vi "NF WF1973_74 OPER Enab.vi"(6 "Read(F)":bool, 8 "error in (no error)":errorcluster caption="Error IN", 9 "Channel(Unavailable)":u16(ring) items=["Unavailable", "Ch1", "Ch2"], 10 "Event Enable(0)":i32(knob) min=0 max=65535 step=1 scale=0.0..65535.0, 11 "VISAsession":refnum<visa-resource-name>) -> (0 "error out":errorcluster caption="Error OUT", 2 "Query Event Enable":i32=99999, 3 "CopyVISAsession":refnum<visa-resource-name>)   [LabVIEW 2010]
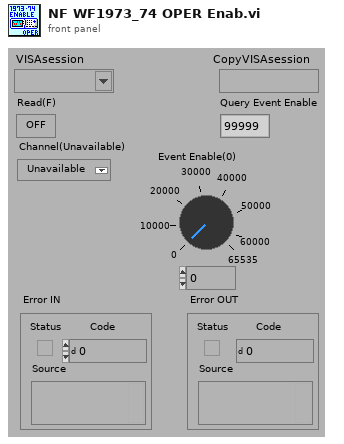
[diagram p1: front panel]
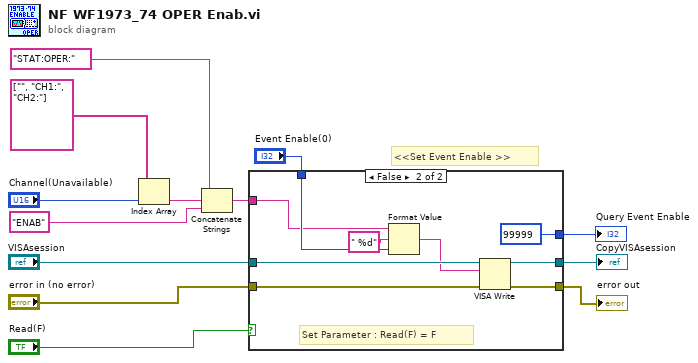
[diagram p0: block diagram]
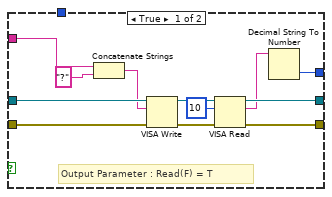
[diagram p2: hidden frame]
diagram:
  # "<<Set Event Enable >>"
  n1 = Index Array(array=string[] ["", "CH1:", "CH2:"], index="Channel(Unavailable)") -> (element=w2:string)
  n2 = Concatenate Strings("STAT:OPER:" ("文字列"), w2, "ENAB" ("文字列")) -> (w4:string)
  n3 = case shown="FALSE" "Read(F)" {
    tunnel: "VISAsession" -> [w25 w34]
    tunnel: [w16 w31] -> w12
    tunnel: [w22 w32] -> w11
    tunnel: "error in (no error)" -> [w21 w33]
    tunnel: w4 -> [w19 w27]
    tunnel: "Event Enable(0)" -> [_ w28]
    tunnel: [w14 99999] -> w7
    frame True {
      # "Output Parameter : Read(F) = T"
      n4 = Concatenate Strings(w19, "?" ("形式文字列")) -> (w17:string)
      n5 = VISA Write(VISA resource name=w25, write buffer=w17, error in (no error)=w21) -> (VISA resource name out=w23:refnum<visa-resource-name>, error out=w24:errorcluster)  [unwired: 1 out]
      n6 = VISA Read(VISA resource name=w23, byte count=u32 10 ("バイトカウント（0）"), error in (no error)=w24) -> (VISA resource name out=w16:refnum<visa-resource-name>, read buffer=w15:string, error out=w22:errorcluster)  [unwired: 1 out]
      n7 = Decimal String To Number(string=w15) -> (number=w14:i32)  [unwired: 2 in, 1 out]
    }
    frame False {
      # "Set Parameter : Read(F) = F"
      n8 = Format Value(string ("")=w27, format string=" %d" ("形式文字列"), value (0)=w28) -> (output string=w26:string)
      n9 = VISA Write(VISA resource name=w34, write buffer=w26, error in (no error)=w33) -> (VISA resource name out=w31:refnum<visa-resource-name>, error out=w32:errorcluster)  [unwired: 1 out]
    }
  }
  "error out" <- w11
  "CopyVISAsession" <- w12
  "Query Event Enable" <- w7
